vi "initialize.vi"(0 "HGF_IMAQDevice":refnum<class "HGF_IMAQDevice.lvclass">, 3 "initializationData":variant, 5 "error in (no error)":errorcluster, 7 "binaryString":string, 8 "I8 Array":i8[](array[numeric]), 9 "prependSize? (T)":bool, 11 "byteOrder (0:big-endian, network order)":T1(ring)) -> (14 "dup HGF_IMAQDevice":refnum<class "HGF_IMAQDevice.lvclass">, 17 "found?":bool, 19 "error out":errorcluster)   [LabVIEW 2014, in "HGF_IMAQ.lvlib" / "HGF_IMAQDevice.lvclass"]
doc: "This is a dynamic dispatch VI to be implemented by child classes to initialize their attributes.\n\n<B>Recommendation:</B> Use Variant for initialization data."
uses:
  HGF_IMAQDevice.lvclass
  HGF_DeviceBaseClasses/HGF_DeviceBase/HGF_DeviceBase.lvclass
  Control Mode.ctl
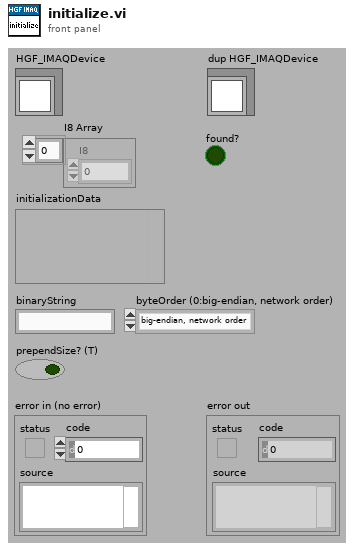
[diagram p1: front panel]
types:
  T1 = enum16{"big-endian, network order", "native, host order", "little-endian"}
  T2 = typedef "Image Type" = u32
  T3 = typedef "HGF_IMAQ.lvlib/HGF_IMAQDevice.lvclass/Control Mode.ctl" = enum16{"Controller", "Listener"}
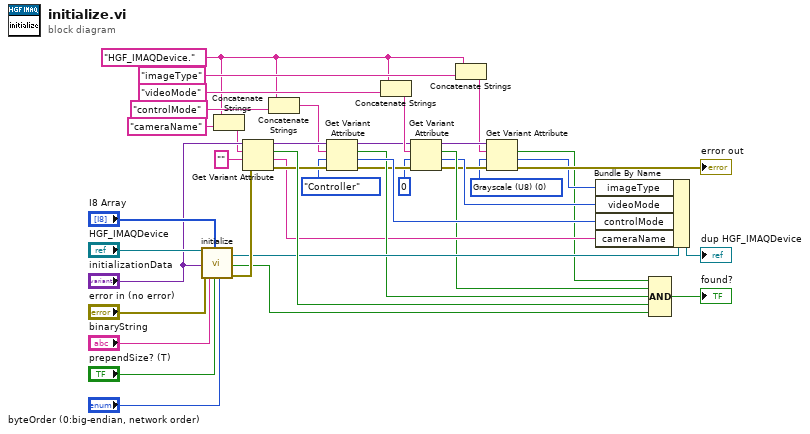
[diagram p0: block diagram]
diagram:
  w3 = T2 0 items=["Grayscale (U8)", "Grayscale (I16)", "Grayscale (SGL)", "Complex (CSG)", "RGB (U32)", "HSL (U32)", "RGB (U64)", "Grayscale (U16)"] ("imageType")
  w8 = "HGF_IMAQDevice." ("name")
  n1 = call-parent "initialize.vi"("HGF_DeviceBase"="HGF_IMAQDevice", "initializationData"="initializationData", "error in (no error)"="error in (no error)", "binaryString"="binaryString", "I8 Array"="I8 Array", "prependSize? (T)"="prependSize? (T)", "byteOrder (0:big-endian, network order)"="byteOrder (0:big-endian, network order)") -> ("dup HGF_DeviceBase"=w29:refnum<class "HGF_IMAQDevice.lvclass">, "found?"=w31:bool, "error out"=w33:errorcluster)  [unwired: 10 out]
  n2 = Concatenate Strings(w8, "cameraName" ("name")) -> (w18:string)
  n3 = Get Variant Attribute(Variant="initializationData", name=w18, default value (empty Variant)="", error in=w33) -> (duplicate Variant=w26:variant, found=w32:bool, value=w15:string, error out=w25:errorcluster)
  n4 = Concatenate Strings(w8, "controlMode" ("name")) -> (w17:string)
  n5 = Get Variant Attribute(Variant=w26, name=w17, default value (empty Variant)=Control_Mode."Controller" ("Control Mode"), error in=w25) -> (duplicate Variant=w13:variant, found=w22:bool, value=w23:T3, error out=w14:errorcluster)
  n6 = Concatenate Strings(w8, "videoMode" ("name")) -> (w16:string)
  n7 = Get Variant Attribute(Variant=w13, name=w16, default value (empty Variant)=0 ("videoMode"), error in=w14) -> (duplicate Variant=w5:variant, found=w12:bool, value=w10:i32, error out=w7:errorcluster)
  n8 = Concatenate Strings(w8, "imageType" ("name")) -> (w4:string)
  n9 = Get Variant Attribute(Variant=w5, name=w4, default value (empty Variant)=w3, error in=w7) -> (found=w1:bool, value=w2:T2, error out=→"error out":errorcluster)  [unwired: 1 out]
  n10 = Bundle By Name(cluster=w29, "imageType"=w2, "videoMode"=w10, "controlMode"=w23, "cameraName"=w15) -> (→"dup HGF_IMAQDevice":refnum<class "HGF_IMAQDevice.lvclass">)
  n11 = Compound Arithmetic op=AND(w1, w12, w22, w32, w31) -> (→"found?":bool)
